vi "ColorListbox.vi"() -> ()   [LabVIEW 2016]
uses:
  <vilib>/Utility/miscctls.llb/LVRowAndColumnTypeDef.ctl
panel:
  out "Array":i32[](array[numeric])
  in  "StatusTable":i32(listbox)
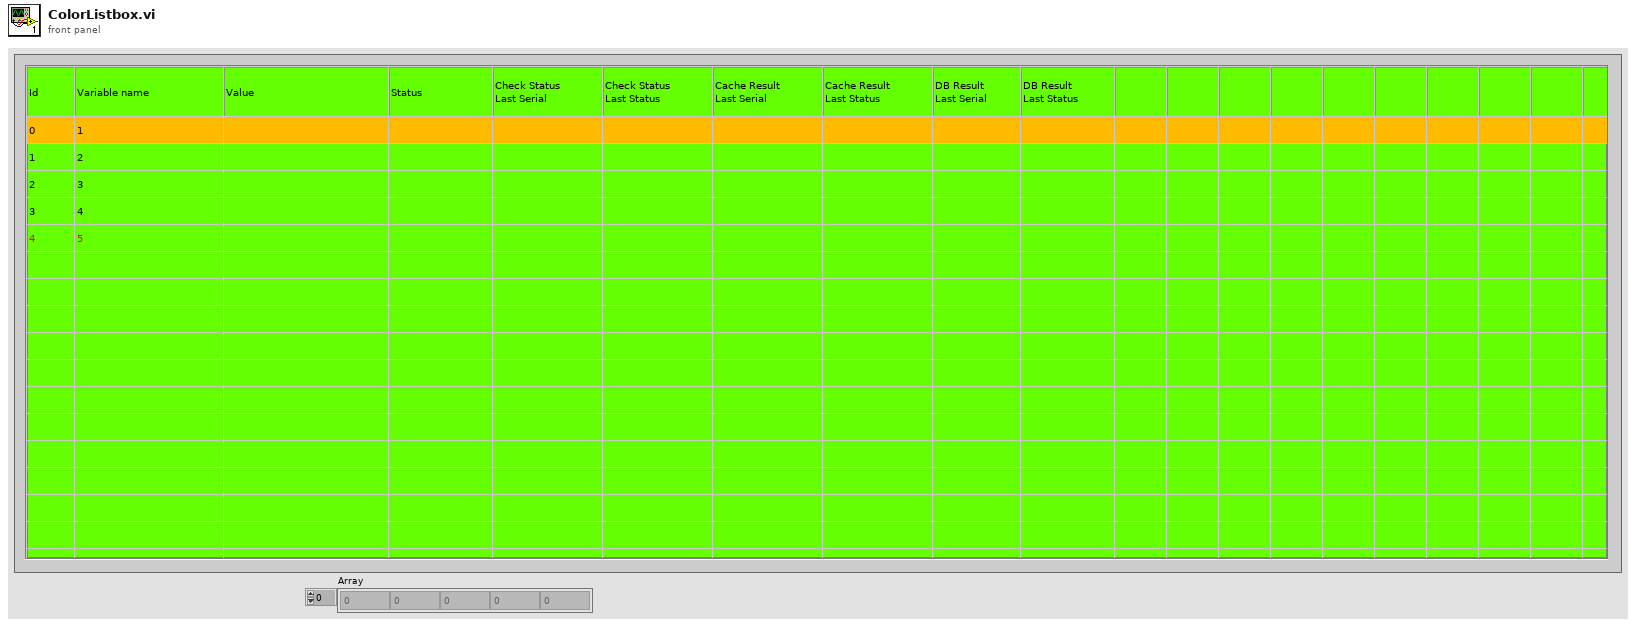
[diagram p1: front panel]
types:
  T1 = typedef "LVRowAndColumnTypeDef.ctl" = cluster{"Row":i32, "Column":i32}
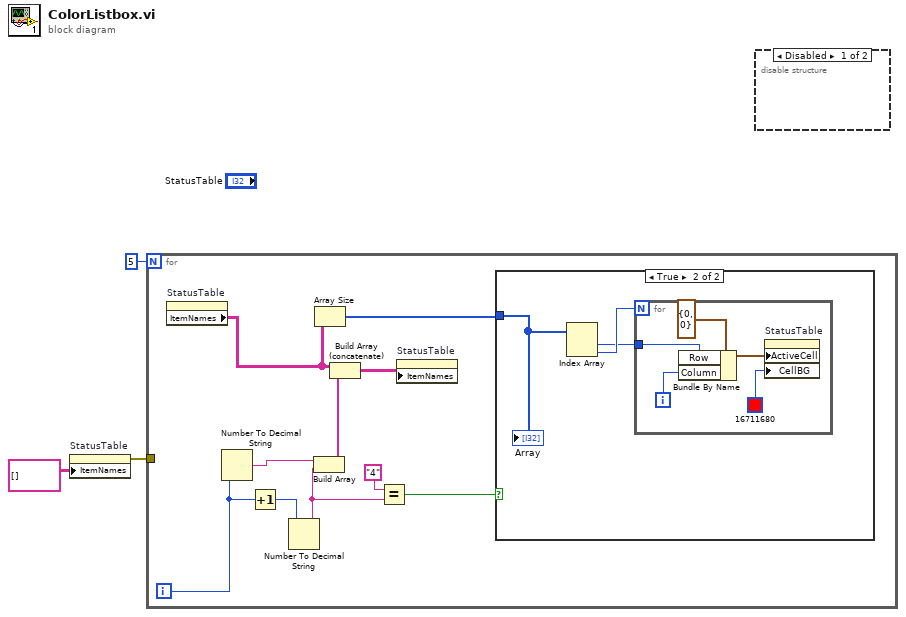
[diagram p0: block diagram]
diagram:
  n1 = property on="StatusTable" class="MCListbox (strict)"("ItemNames"=string[][] [] ("Item Names")) -> (error out=w2:errorcluster)  [unwired: 2 in, 1 out]
  n2 = for {
    N: 5 -> [_]
    tunnel: w2 -> [_]
    i -> [w10]
    n3 = property on="StatusTable" class="MCListbox (strict)"() -> ("ItemNames"=w6:string[][])  [unwired: 2 in, 2 out]
    n4 = Number To Decimal String(number=w10) -> (decimal integer string=w12:string)  [unwired: 1 in]
    n5 = Increment(x=w10) -> (x+1=w9:i32)
    n6 = Number To Decimal String(number=w9) -> (decimal integer string=w8:string)  [unwired: 1 in]
    n7 = Build Array(w12, w8) -> (w11:string[])
    n8 = Array Size(array=w6) -> (size(s)=w4:i32[])
    n9 = Build Array (concatenate)(w6, w11) -> (w13:string[][])
    n10 = Equal?(x="4", y=w8) -> (x = y?=w5:bool)
    n11 = property on="StatusTable" class="MCListbox (strict)"("ItemNames"=w13) -> ()  [unwired: 2 in, 2 out]
    n12 = case shown="True" w5 {
      tunnel: w4 -> [_ w16]
      frame False {
      }
      frame True {
        n13 = Index Array(array=w16) -> (element #1=w14:i32, element #2=w15:i32)  [unwired: 2 in]
        n14 = for {
          N: w15 -> [_]
          tunnel: w14 -> [w17]
          i -> [w20]
          n15 = Bundle By Name(cluster=T1 {"Row"=0, "Column"=0} ("Active Cell:Active Cell"), "Row"=w17, "Column"=w20) -> (w19:T1)
          n16 = property on="StatusTable" class="MCListbox (strict)"("ActiveCell"=w19, "CellBG"=u32 16711680) -> ()  [unwired: 2 in, 2 out]
        }
        "Array" <- w16
      }
    }
  }
  n17 = disable-structure shown="Disabled" {
    frame Disabled {
    }
    frame Enabled {
    }
  }
